vi "Configuration.vi"(6 "Return Data":refnum<user-event>, 8 "error in (no error)":errorcluster, 9 "Exit Running Config":refnum<user-event>, 10 "Panel in":refnum<class "Panel.lvclass">, 11 "String Data Type in":refnum<class "String Data Type.lvclass">) -> (0 "error out":errorcluster, 3 "String Data Type out":refnum<class "String Data Type.lvclass">)   [LabVIEW 2018, in "String Data Type.lvclass"]
uses:
  String Data Type.lvclass
  D:/Code/QControls Extended/DataGrid/DataGrid Configuration/Data Type Classes/Generic/Generic Data Type.lvclass
  <vilib>/MGI/Panel Manager/Panel/Panel/Panel.lvclass
  Generic/Generic Data Type.lvclass
  Display Style Enum.ctl
  String Data Type.lvclass/String Data Type.ctl
  Generic/Generic Data Type.lvclass/Generic Data Type.ctl
  Generic/Write Column Header.vi
  Generic/Read Column Header.vi
panel:
  in  "Column Header":string
  in  "Default Value":string
  in  "Display Style":T1
  # "String Column"
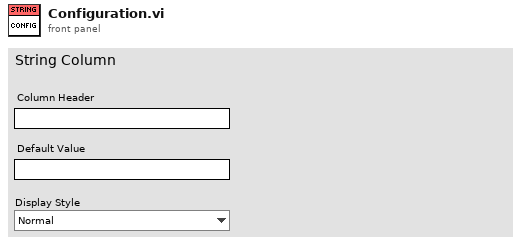
[diagram p1: front panel]
types:
  T1 = typedef "String Data Type.lvclass/Display Style Enum.ctl" = enum16{"Normal", "'\\' Codes", "Hex"}
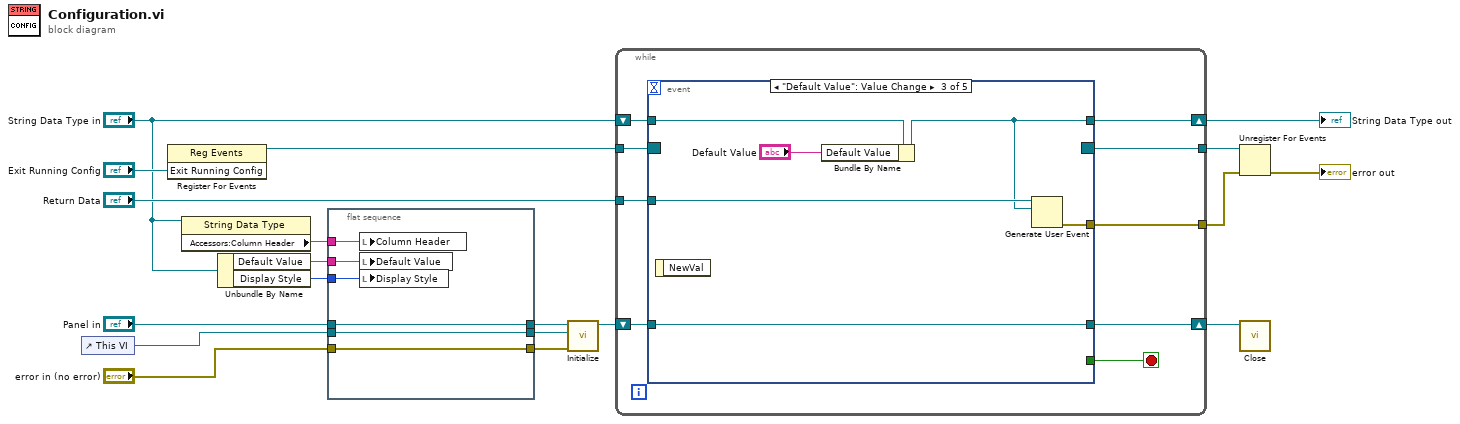
[diagram p0: block diagram]
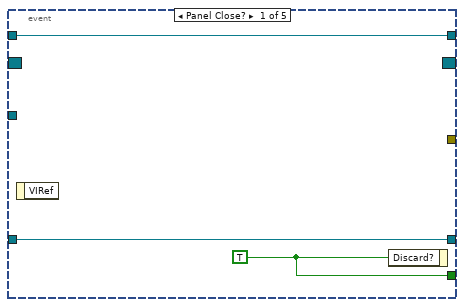
[diagram p2: hidden frame]
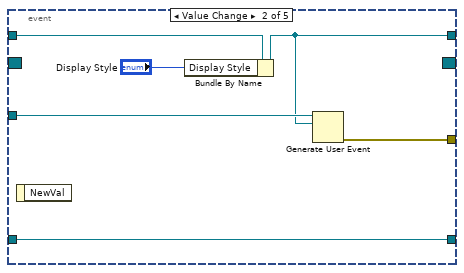
[diagram p3: hidden frame]
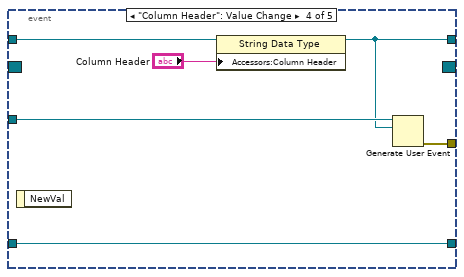
[diagram p4: hidden frame]
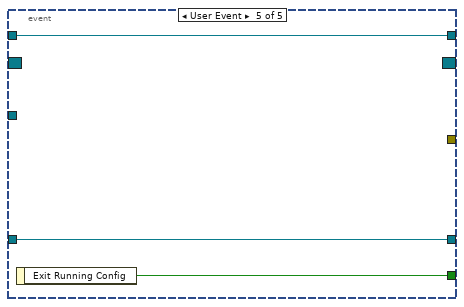
[diagram p5: hidden frame]
diagram:
  n1 = control-ref of="This VI"() -> (w7:refnum<vi>)
  n2 = register-events("Exit Running Config") -> (reference out=w18:refnum<event-registration>)  [unwired: 2 in, 1 out]
  n3 = property class="String Data Type"(reference="String Data Type in") -> ("Accessors:Column Header"=w1:string)  [unwired: 1 in, 2 out]
  n4 = Unbundle By Name("String Data Type in") -> ("Default Value"=w3:string, "Display Style"=w11:T1)
  n5 = flat-sequence {
    tunnel: w11 -> [w25]
    tunnel: "Panel in" -> [w24]
    tunnel: [w24] -> w9
    tunnel: [w23] -> w8
    tunnel: w7 -> [w23]
    tunnel: "error in (no error)" -> [w22]
    tunnel: [w22] -> w4
    tunnel: w3 -> [w21]
    tunnel: w1 -> [w20]
    frame #0 {
      n6 = local write "Column Header"(w20) -> ()
      n7 = local write "Default Value"(w21) -> ()
      n8 = local write "Display Style"(w25) -> ()
    }
  }
  n9 = call <vilib>:"Initialize.vi"("error in (no error)"=w4, "VI Refnum"=w8, "Panel In"=w9) -> ("Panel Out"=w16:refnum<class "Panel.lvclass">)  [unwired: 6 in, 2 out]
  n10 = while {
    shift-right: [w28] -> w15
    shift-left: "String Data Type in" -> [w34]
    shift-right: [w30] -> w17
    shift-left: w16 -> [w31]
    tunnel: w18 -> [w32]
    tunnel: [w29] -> w19
    tunnel: "Return Data" -> [w27]
    tunnel: [w26] -> w6
    stop <- w33 stop-if-true
    n11 = event shown="[2] \"Default Value\": Value Change" {
      selector: w32 -> [_ _ _ _ _]
      dyn-events: [_ _ _ _ _] -> w29
      timeout: _ -> [_ _ _ _ _]
      tunnel: w34 -> [w37 w42 w48 w52 w58]
      tunnel: [w37 w39 w46 w51 w58] -> w28
      tunnel: [w36 _ _ _ w57] -> w33
      tunnel: w31 -> [w35 w43 w49 w55 w56]
      tunnel: [w35 w43 w49 w55 w56] -> w30
      tunnel: w27 -> [_ w40 w47 w54 _]
      tunnel: [_ w38 w45 w53 _] -> w26
      event Panel Close? {
        w36 = TRUE
        n12 = event-data() -> ()  [unwired: 1 in, 1 out]
        n13 = event-data("Discard?"=w36) -> ()  [unwired: 1 in, 1 out]
      }
      event Value Change {
        n14 = event-data() -> ()  [unwired: 1 in, 1 out]
        n15 = Bundle By Name(cluster=w42, "Display Style"="Display Style") -> (w39:refnum<class "String Data Type.lvclass">)
        n16 = Generate User Event(user event=w40, event data cluster=w39) -> (error out=w38:errorcluster)  [unwired: 2 in, 1 out]
      }
      event "Default Value": Value Change {
        n17 = event-data() -> ()  [unwired: 1 in, 1 out]
        n18 = Bundle By Name(cluster=w48, "Default Value"="Default Value") -> (w46:refnum<class "String Data Type.lvclass">)
        n19 = Generate User Event(user event=w47, event data cluster=w46) -> (error out=w45:errorcluster)  [unwired: 2 in, 1 out]
      }
      event "Column Header": Value Change {
        n20 = event-data() -> ()  [unwired: 1 in, 1 out]
        n21 = property class="String Data Type"(reference=w52, "Accessors:Column Header"="Column Header") -> (reference out=w51:refnum<class "String Data Type.lvclass">)  [unwired: 1 in, 1 out]
        n22 = Generate User Event(user event=w54, event data cluster=w51) -> (error out=w53:errorcluster)  [unwired: 2 in, 1 out]
      }
      event User Event {
        n23 = event-data() -> ("Exit Running Config"=w57:bool)  [unwired: 1 in]
      }
    }
  }
  "String Data Type out" <- w15
  n24 = Unregister For Events(event registration refnum=w19, error in=w6) -> (error out=→"error out":errorcluster)
  n25 = call-dynamic "Close.vi"("Panel In"=w17) -> ()  [unwired: 10 in, 1 out]
